vi "11. SCADA_Bottle_Filling_2.vi"() -> ()   [LabVIEW 2020]
panel:
  in  "Valve":bool
  in  "Slide":dbl(slide) scale=0.0..1000.0
  out "Valve":bool
  out "Water_Upper":dbl(slide) scale=650.0..543.0
  out "Water_Down":dbl(slide)
  out "Bottle_1":dbl(slide) scale=548.0..600.0
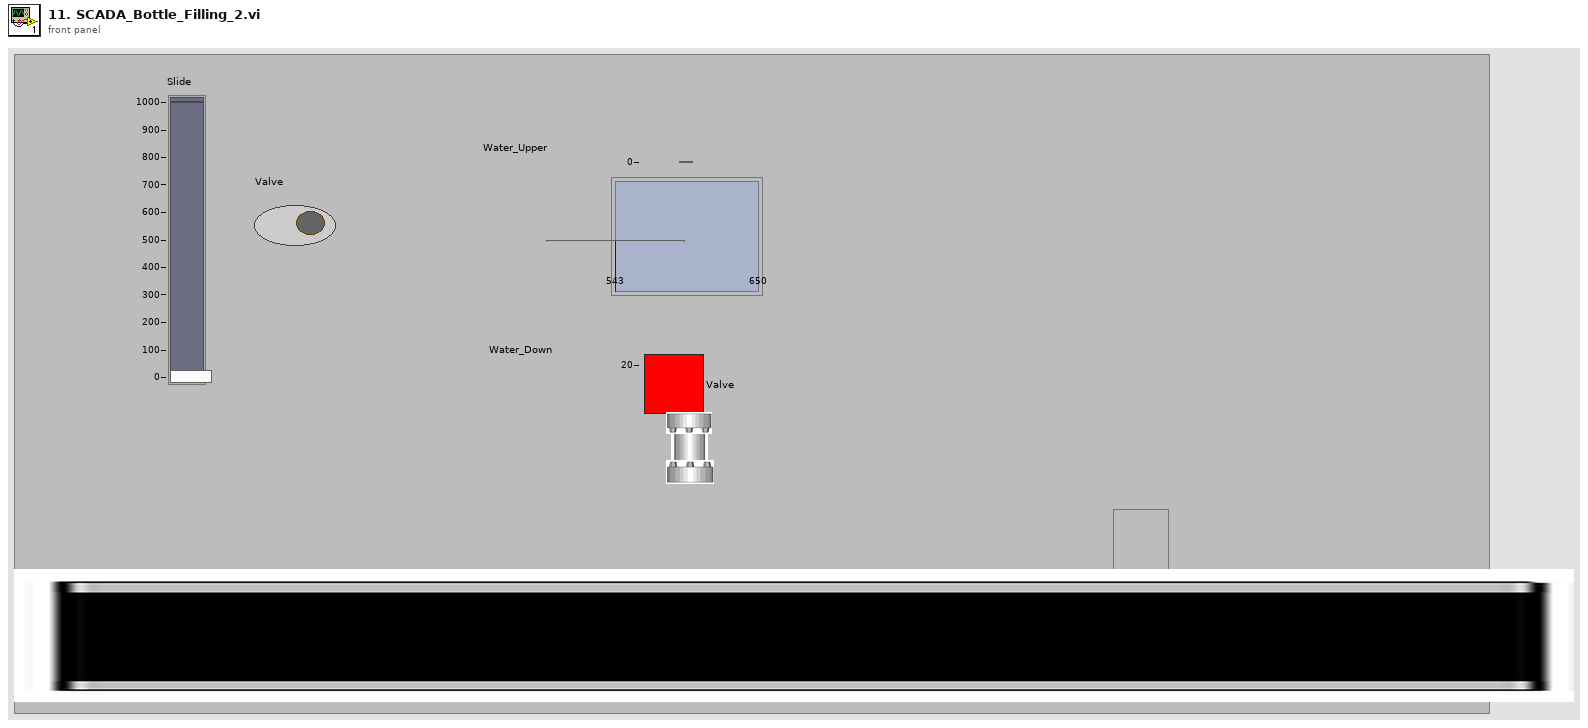
[diagram p1: front panel]
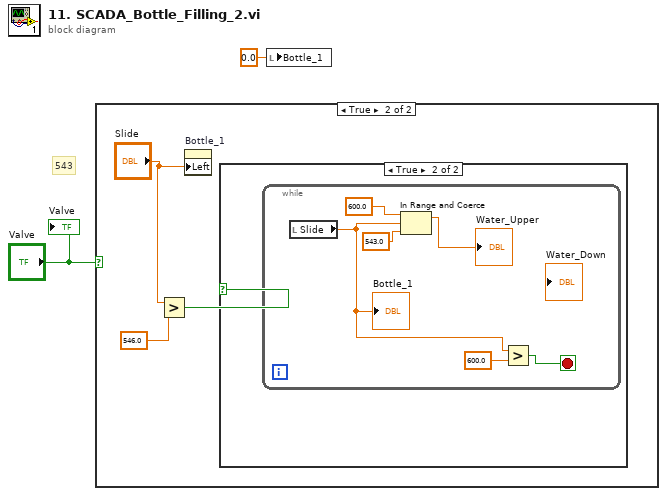
[diagram p0: block diagram]
diagram:
  # "543"
  n1 = case shown="True" "Valve" {
    frame False {
    }
    frame True {
      n2 = Greater?(x="Slide", y=546.0) -> (0:w5:bool)
      n3 = property on="Bottle_1" class="Slide (strict)"("Left"="Slide") -> ()  [unwired: 2 in, 2 out]
      n4 = case shown="True" w5 {
        frame False {
        }
        frame True {
          n5 = while {
            stop <- w10 stop-if-true
            n6 = local read "Slide"() -> (w9:dbl)
            "Bottle_1" <- w9
            n7 = In Range and Coerce(upper limit=600.0, x=w9, lower limit=543.0) -> (coerced(x)=→"Water_Upper":dbl)  [unwired: 1 out]
            n8 = Greater?(x=w9, y=600.0) -> (0:w10:bool)
          }
        }
      }
    }
  }
  n9 = local write "Bottle_1"(0.0 ("Bottle_1")) -> ()
  "Valve" <- "Valve"
